vi "Keithley Sample Number.vi"(9 "Step":dbl=2.0, 10 "Stop":dbl=2.0, 11 "Start":dbl=1.0) -> (2 "Array":dbl[](array[numeric]) format="%#.1f", 3 "pointnumber":dbl)   [LabVIEW 2017]
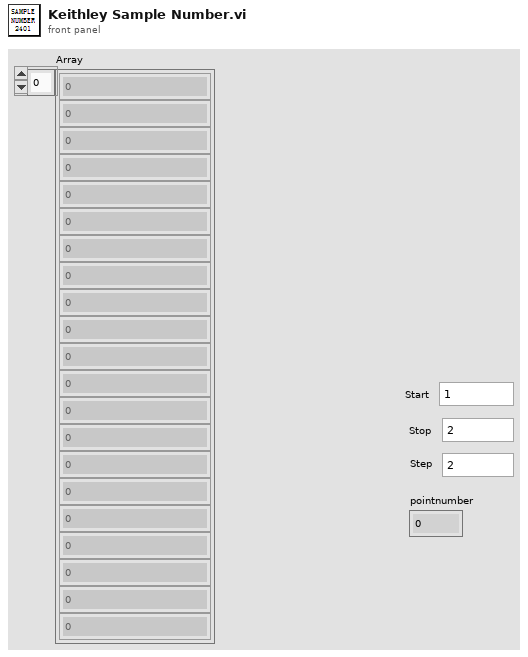
[diagram p1: front panel]
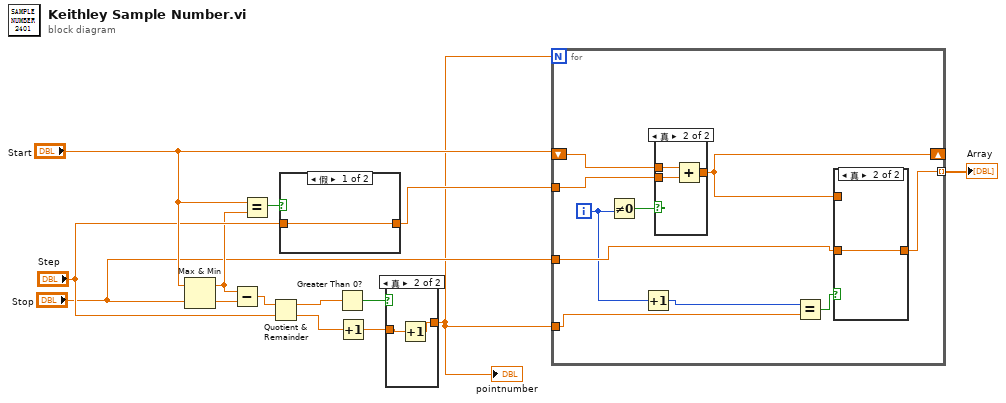
[diagram p0: block diagram]
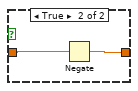
[diagram p3: hidden frame]
diagram:
  n1 = Max & Min(x="Start", y="Stop") -> (max(x,y)=w4:dbl, min(x,y)=w13:dbl)
  n2 = Subtract(x=w4, y=w13) -> (x-y=w14:dbl)
  n3 = Equal?(x="Start", y=w4) -> (x = y?=w11:bool)
  n4 = Quotient & Remainder(x=w14, y="Step") -> (x-y*floor(x/y)=w8:dbl, floor(x/y)=w6:dbl)
  n5 = case shown="假" w11 {
    tunnel: "Step" -> [w15 w17]
    tunnel: [w15 w16] -> w9
    frame False {
    }
    frame True {
      n6 = Negate(x=w17) -> (-x=w16:dbl)
    }
  }
  n7 = Greater Than 0?(x=w8) -> (x > 0?=w7:bool)
  n8 = Increment(x=w6) -> (x+1=w5:dbl)
  n9 = case shown="真" w7 {
    tunnel: [w18 w19] -> w1
    tunnel: w5 -> [w18 w20]
    frame False {
    }
    frame True {
      n10 = Increment(x=w20) -> (x+1=w19:dbl)
    }
  }
  "pointnumber" <- w1
  n11 = for {
    N: w1 -> [_]
    tunnel: w9 -> [w29]
    shift-right: [w26] -> _
    shift-left: "Start" -> [w30]
    tunnel: "Stop" -> [w25]
    tunnel: [w27] -> w3 mode=indexing
    tunnel: w1 -> [w22]
    i -> [w24]
    n12 = Not Equal To 0?(x=w24) -> (x != 0?=w28:bool)
    n13 = Increment(x=w24) -> (x+1=w23:i32)
    n14 = case shown="真" w28 {
      tunnel: w30 -> [w33 w36]
      tunnel: w29 -> [_ w35]
      tunnel: [w33 w34] -> w26
      frame False {
      }
      frame True {
        n15 = Add(x=w36, y=w35) -> (x+y=w34:dbl)
      }
    }
    n16 = Equal?(x=w23, y=w22) -> (x = y?=w21:bool)
    n17 = case shown="真" w21 {
      tunnel: w25 -> [_ w32]
      tunnel: [w31 w32] -> w27
      tunnel: w26 -> [w31 _]
      frame False {
      }
      frame True {
      }
    }
  }
  "Array" <- w3
